vi "GE 5565PIORC.DMA.Create Transfer (multiple).vi"(8 "error in (no error)":errorcluster, 9 "RFM offset":u32, 10 "Block Descriptors":T2[](array[typedef]) {"next descriptor ptr" format="%08x"; "data size" format="%08x"; "data ptr (upper)" format="%08x"; "data ptr (lower)" format="%08x"; "descriptor ptr (aligned)" format="%08x"; "descriptor size" format="%08x"; "descriptor ptr (VISA)" format="%08x"}, 11 "GE 5565PIORC in":refnum<class "GE 5565PIORC.lvclass">) -> (0 "error out":errorcluster, 1 "transfer size (bytes)":u32, 2 "DMA Transfer Spec":T1 {"Block Descriptors"."next descriptor ptr" format="%08x"; "Block Descriptors"."data size" format="%08x"; "Block Descriptors"."data ptr (upper)" format="%08x"; "Block Descriptors"."data ptr (lower)" format="%08x"; "Block Descriptors"."descriptor ptr (aligned)" format="%08x"; "Block Descriptors"."descriptor size" format="%08x"; "Block Descriptors"."descriptor ptr (VISA)" format="%08x"; "RFM offset" format="%08x"}, 3 "GE 5565PIORC out":refnum<class "GE 5565PIORC.lvclass">)   [LabVIEW 2016, in "GE 5565PIORC.lvclass"]
doc: "Creates a <B>DMA Transfer Spec</B> which associates a series of <B>Block Descriptors</B> to an offset in Reflective Memory."
uses:
  GE 5565PIORC.lvclass
  Typedefs/GE 5565PIORC.Typdef.DMA Block Descriptor.ctl
  Typedefs/GE 5565PIORC.Typdef.DMA Transfer Spec.ctl
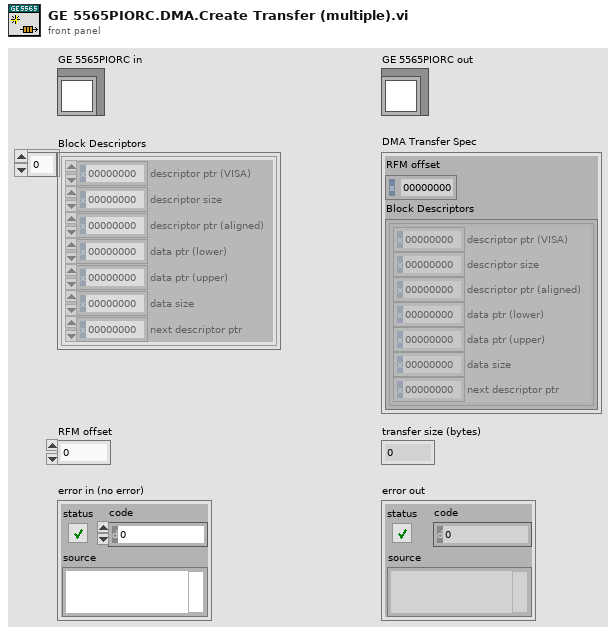
[diagram p1: front panel]
types:
  T1 = typedef "GE 5565PIORC.lvclass/GE 5565PIORC.Typdef.DMA Transfer Spec.ctl" = cluster{"RFM offset":u32, "Block Descriptors":T2[]}
  T2 = typedef "GE 5565PIORC.lvclass/GE 5565PIORC.Typdef.DMA Block Descriptor.ctl" = cluster{"descriptor ptr (VISA)":u32, "descriptor size":u32, "descriptor ptr (aligned)":u32, "data ptr (lower)":u32, "data ptr (upper)":u32, "data size":u32, "next descriptor ptr":u32}
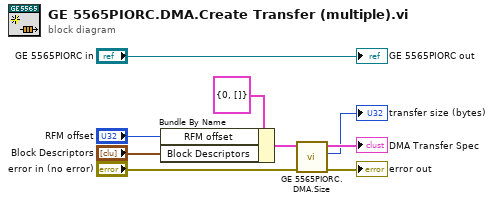
[diagram p0: block diagram]
diagram:
  n1 = Bundle By Name(cluster=T1 {"RFM offset"=0, "Block Descriptors"=[]} ("DMA Transfer Spec"), "RFM offset"="RFM offset", "Block Descriptors"="Block Descriptors") -> (w7:T1)
  n2 = call "GE 5565PIORC.DMA.Size.vi"("error in (no error)"="error in (no error)", "DMA Transfer Spec in"=w7) -> ("error out"=→"error out":errorcluster, "transfer size (bytes)"=→"transfer size (bytes)":u32, "DMA Transfer Spec out"=→"DMA Transfer Spec":T1)  [unwired: 7 in]
  "GE 5565PIORC out" <- "GE 5565PIORC in"
